vi "SERVREST_POST.vi"(6 "error in":errorcluster, 7 "pwd":string, 8 "User":string, 9 "JSON Object":string, 10 "x-nem-datetime":string, 11 "URL":string) -> (0 "error out":errorcluster, 2 "Response JSON":string, 3 "Response headers":string)   [LabVIEW 2015]
uses:
  <vilib>/httpClient/POSTBuffer.vi
  <vilib>/httpClient/LabVIEWHTTPClient.lvlib
  AURA_Wheel/AuraWheelAPI/AuraWheel.lvlib
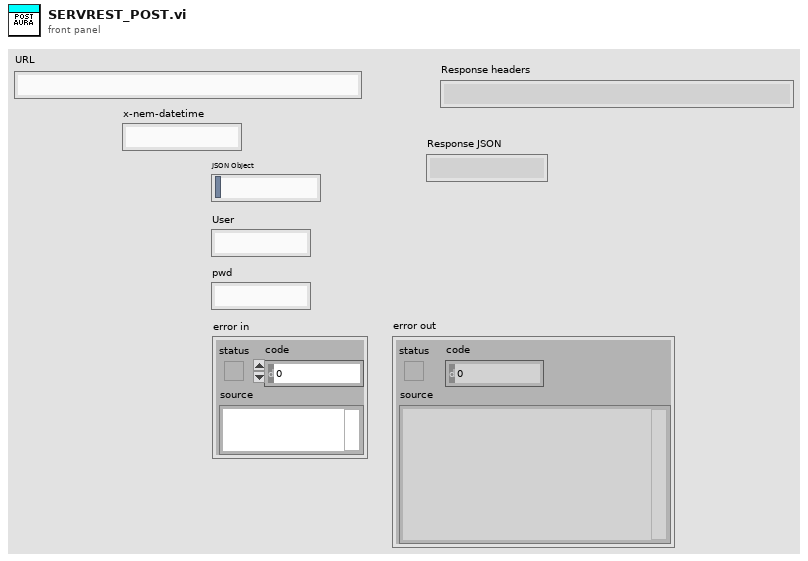
[diagram p1: front panel]
types:
  T1 = typedef "LabVIEWHTTPClient.lvlib/ClientHandle.ctl" = refnum<k1>
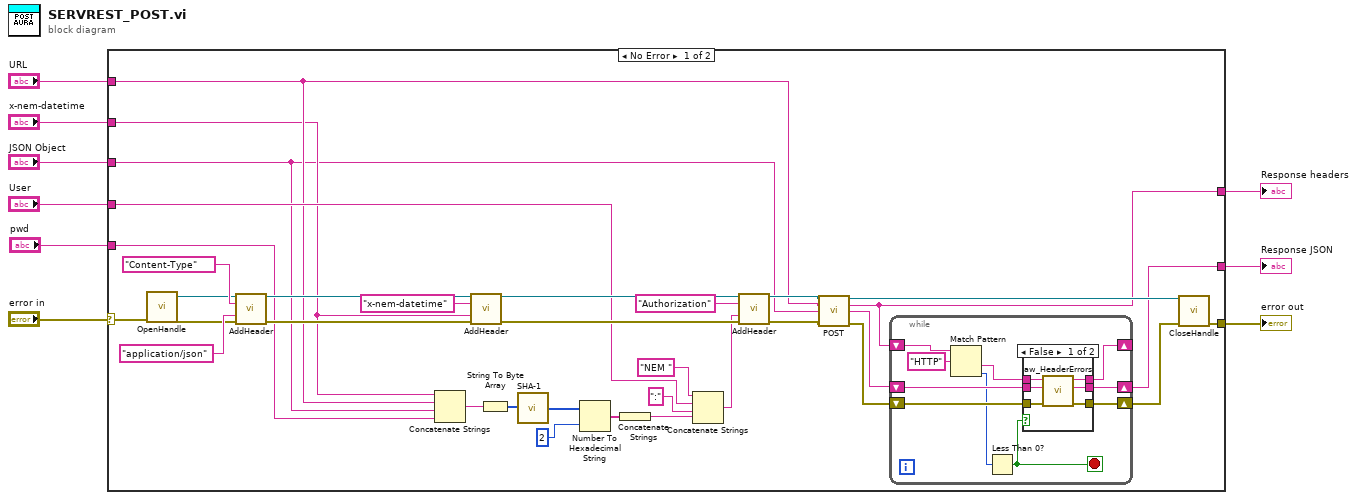
[diagram p0: block diagram]
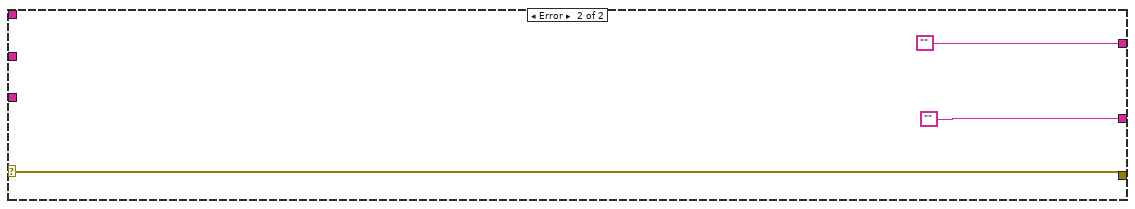
[diagram p3: hidden frame]
diagram:
  n1 = case shown="No Error" "error in" {
    selector: "error in" -> [w29 w65]
    tunnel: "x-nem-datetime" -> [w14 _]
    tunnel: [w28 w65] -> w7
    tunnel: "URL" -> [w17 _]
    tunnel: "JSON Object" -> [w11 _]
    tunnel: "pwd" -> [w21 _]
    tunnel: [w10 ""] -> w3
    tunnel: [w12 ""] -> w2
    tunnel: "User" -> [w20 _]
    frame No Error {
      n2 = call <vilib>:"OpenHandle.vi"("error in (no error)"=w29) -> ("client handle out"=w31:T1, "error out"=w32:errorcluster)  [unwired: 13 in]
      n3 = call <vilib>:"AddHeader.vi"("client handle"=w31, "header"="Content-Type", "value"="application/json", "error in (no error)"=w32) -> ("client handle out"=w43:T1, "error out"=w42:errorcluster)  [unwired: 10 in]
      n4 = Concatenate Strings(w14, w17, w11, w21) -> (w37:string)
      n5 = call <vilib>:"AddHeader.vi"("client handle"=w43, "header"="x-nem-datetime" ("value"), "value"=w14, "error in (no error)"=w42) -> ("client handle out"=w40:T1, "error out"=w39:errorcluster)  [unwired: 10 in]
      n6 = String To Byte Array(string=w37) -> (unsigned byte array=w36:u8[])
      n7 = call "SHA-1.vi"("Data"=w36) -> ("message-digest"=w35:u8[])
      n8 = Number To Hexadecimal String(1:i16 2 ("width (-)"), 2:w35) -> (0:w34:string[])
      n9 = Concatenate Strings(w34) -> (w27:string)
      n10 = Concatenate Strings("NEM " ("string"), w20, ":" ("string"), w27) -> (w26:string)
      n11 = call <vilib>:"AddHeader.vi"("client handle"=w40, "header"="Authorization" ("value"), "value"=w26, "error in (no error)"=w39) -> ("client handle out"=w18:T1, "error out"=w16:errorcluster)  [unwired: 10 in]
      n12 = call-poly <vilib>:"POST.vi"("client handle"=w18, "url"=w17, "buffer"=w11, "error in (no error)"=w16) -> ("client handle out"=w19:T1, "headers"=w10:string, "body"=w13:string, "error out"=w15:errorcluster)  [unwired: 8 in]
      n13 = while {
        shift-right: [w53] -> w24
        shift-left: w15 -> [w52]
        shift-right: [w49] -> _
        shift-left: w10 -> [w47]
        shift-right: [w46] -> w12
        shift-left: w13 -> [w50]
        stop <- w44 stop-if-true
        n14 = Match Pattern(string=w47, regular expression="HTTP") -> (after substring=w51:string, offset past match=w45:i32)  [unwired: 1 in, 2 out]
        n15 = Less Than 0?(x=w45) -> (x < 0?=w44:bool)
        n16 = case shown="False" w44 {
          tunnel: [w59 w60] -> w53
          tunnel: w52 -> [w58 w60]
          tunnel: w51 -> [w57 w62]
          tunnel: w50 -> [w56 w61]
          tunnel: [w55 w62] -> w49
          tunnel: [w54 w61] -> w46
          frame False {
            n17 = call "aw_HeaderErrors.vi"("error in"=w58, "Response Body"=w56, "Response Headers"=w57) -> ("error out"=w59:errorcluster, "Response Body Out"=w54:string, "Response Headers Out"=w55:string)  [unwired: 6 in]
          }
          frame True {
          }
        }
      }
      n18 = call <vilib>:"CloseHandle.vi"("client handle"=w19, "error in (no error)"=w24) -> ("error out"=w28:errorcluster)  [unwired: 13 in]
    }
    frame Error {
    }
  }
  "error out" <- w7
  "Response headers" <- w3
  "Response JSON" <- w2
